vi "Chack Motor.vi"(11 "Input V70 Values":string) -> (0 "Low":string, 1 "High":string, 2 "Diff":string, 3 "diffAllowed":string, 4 "Result Motor Performance":string, 5 "Step Remark":string, 6 "error out":errorcluster, 7 "Status":bool)   [LabVIEW 2020, in "FBN_LATM.lvlib"]
uses:
  FBN_LATM.lvlib
  <vilib>/regexp/Match Regular Expression.xnode
panel:
  out "spreadsheet string":string
  out "Greater Than":bool
  out "OK?":bool
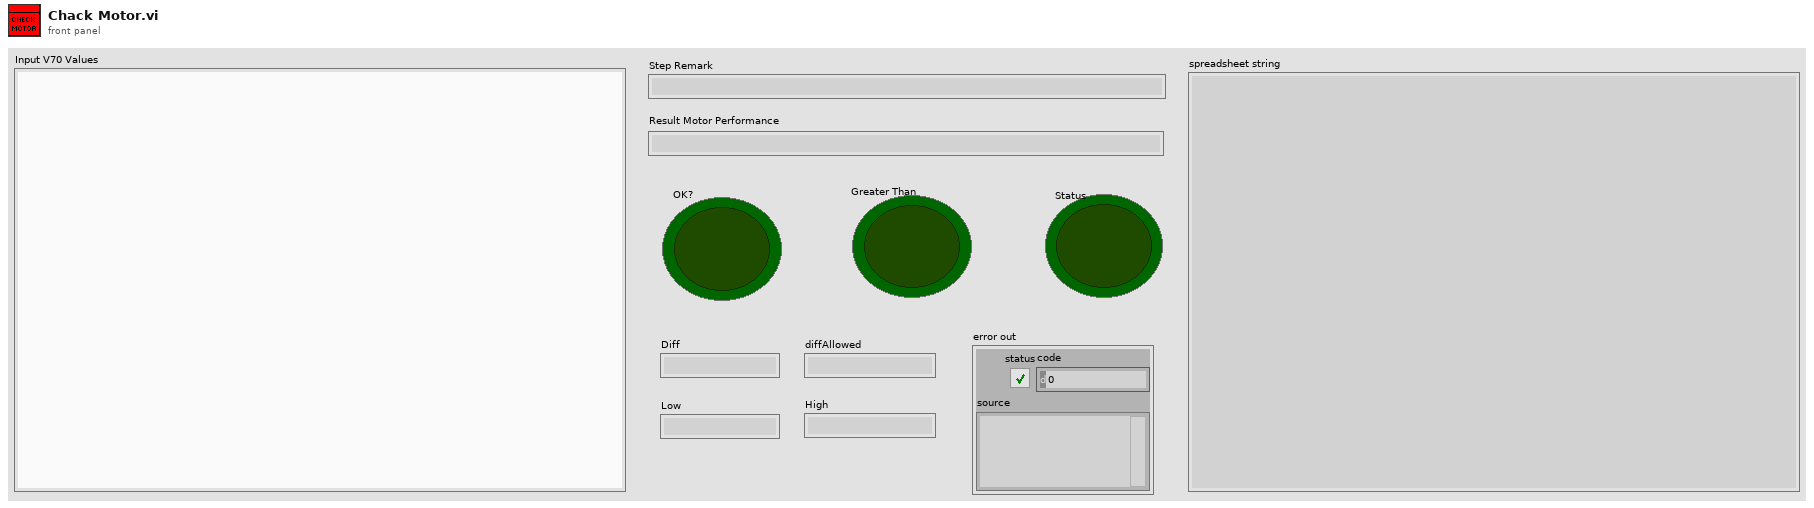
[diagram p1: front panel]
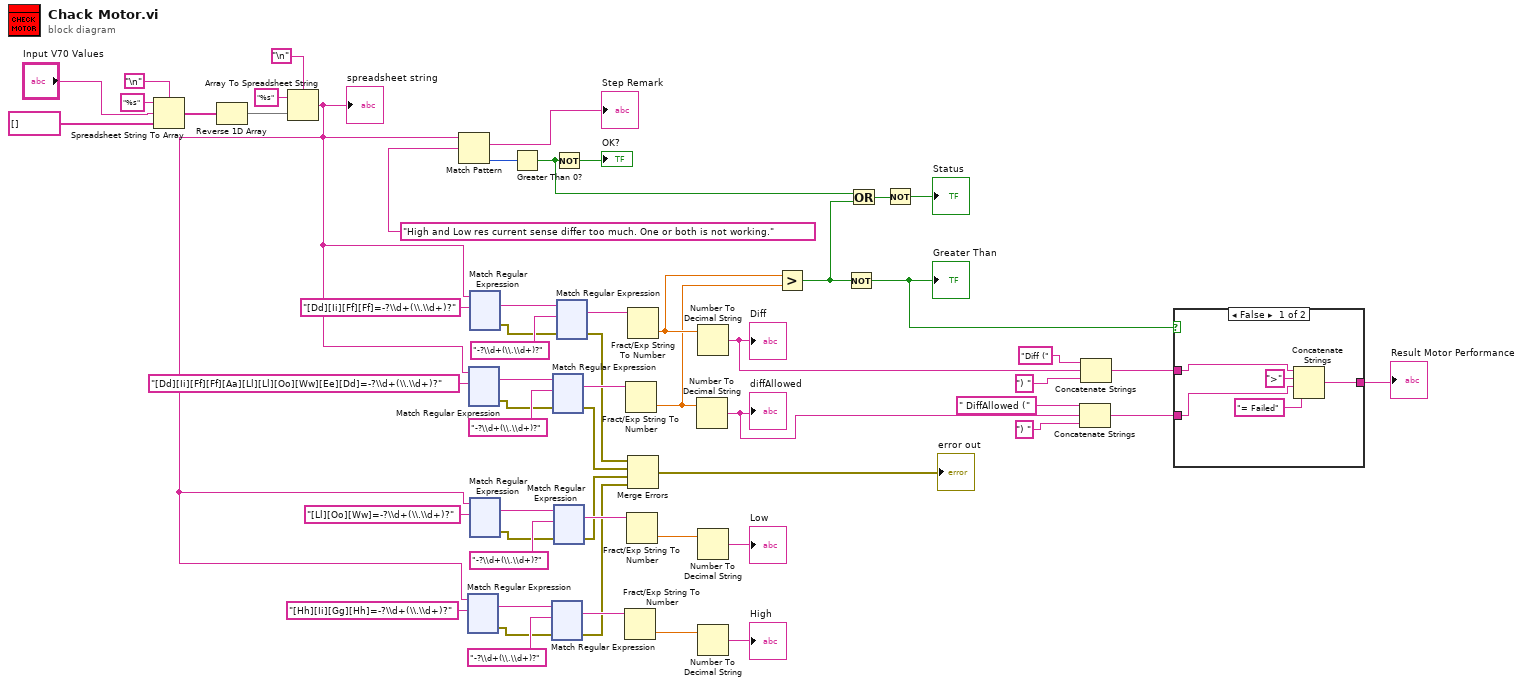
[diagram p0: block diagram]
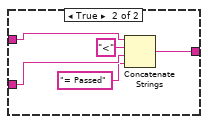
[diagram p2: hidden frame]
diagram:
  n1 = Spreadsheet String To Array(delimiter (Tab)="\n", format string="%s", spreadsheet string="Input V70 Values", array type (2D Dbl)=string[] []) -> (array=w17:string[])
  n2 = Reverse 1D Array(array=w17) -> (reversed array=w13:string[])
  n3 = Array To Spreadsheet String(delimiter (Tab)="\n", array=w13, 3:"%s" ("format string")) -> (spreadsheet string=w12:string)
  "spreadsheet string" <- w12
  n4 = Match Pattern(string=w12, regular expression="High and Low res current sense differ too much. One or both is not working.") -> (match substring=→"Step Remark":string, offset past match=w57:i32)  [unwired: 1 in, 2 out]
  n5 = xnode "Match Regular Expression"("input string"=w12, "regular expression"="[Hh][Ii][Gg][Hh]=-?\\d+(\\.\\d+)?") -> ("whole match"=w30:string, "error out"=w29:errorcluster)  [unwired: 4 in, 3 out]
  n6 = xnode "Match Regular Expression"("input string"=w12, "regular expression"="[Dd][Ii][Ff][Ff][Aa][Ll][Ll][Oo][Ww][Ee][Dd]=-?\\d+(\\.\\d+)?") -> ("whole match"=w48:string, "error out"=w46:errorcluster)  [unwired: 4 in, 3 out]
  n7 = xnode "Match Regular Expression"("input string"=w12, "regular expression"="[Dd][Ii][Ff][Ff]=-?\\d+(\\.\\d+)?") -> ("whole match"=w53:string, "error out"=w47:errorcluster)  [unwired: 4 in, 3 out]
  n8 = xnode "Match Regular Expression"("input string"=w12, "regular expression"="[Ll][Oo][Ww]=-?\\d+(\\.\\d+)?") -> ("whole match"=w35:string, "error out"=w34:errorcluster)  [unwired: 4 in, 3 out]
  n9 = Greater Than 0?(x=w57) -> (x > 0?=w40:bool)
  n10 = xnode "Match Regular Expression"("input string"=w30, "regular expression"="-?\\d+(\\.\\d+)?", "error in"=w29) -> ("whole match"=w31:string, "error out"=w27:errorcluster)  [unwired: 3 in, 3 out]
  n11 = xnode "Match Regular Expression"("input string"=w48, "regular expression"="-?\\d+(\\.\\d+)?", "error in"=w46) -> ("whole match"=w49:string, "error out"=w44:errorcluster)  [unwired: 3 in, 3 out]
  n12 = Not(x=w40) -> (.not. x?=→"OK?":bool)
  n13 = xnode "Match Regular Expression"("input string"=w35, "regular expression"="-?\\d+(\\.\\d+)?", "error in"=w34) -> ("whole match"=w36:string, "error out"=w28:errorcluster)  [unwired: 3 in, 3 out]
  n14 = xnode "Match Regular Expression"("input string"=w53, "regular expression"="-?\\d+(\\.\\d+)?", "error in"=w47) -> ("whole match"=w51:string, "error out"=w45:errorcluster)  [unwired: 3 in, 3 out]
  n15 = Fract/Exp String To Number(string=w31) -> (number=w22:dbl)  [unwired: 3 in, 1 out]
  n16 = Fract/Exp String To Number(string=w49) -> (number=w25:dbl)  [unwired: 3 in, 1 out]
  n17 = Fract/Exp String To Number(string=w36) -> (number=w21:dbl)  [unwired: 3 in, 1 out]
  n18 = Fract/Exp String To Number(string=w51) -> (number=w26:dbl)  [unwired: 3 in, 1 out]
  n19 = Merge Errors(w45, w44, w28, w27) -> (→"error out":errorcluster)
  n20 = Number To Decimal String(number=w25) -> (decimal integer string=w5:string)  [unwired: 1 in]
  "diffAllowed" <- w5
  n21 = Number To Decimal String(number=w26) -> (decimal integer string=w10:string)  [unwired: 1 in]
  "Diff" <- w10
  n22 = Number To Decimal String(number=w21) -> (decimal integer string=→"Low":string)  [unwired: 1 in]
  n23 = Number To Decimal String(number=w22) -> (decimal integer string=→"High":string)  [unwired: 1 in]
  n24 = Greater?(x=w26, y=w25) -> (0:w39:bool)
  n25 = Not(x=w39) -> (.not. x?=w1:bool)
  "Greater Than" <- w1
  n26 = Or(x=w40, y=w39) -> (x .or. y?=w41:bool)
  n27 = Not(x=w41) -> (.not. x?=→"Status":bool)
  n28 = Concatenate Strings(" DiffAllowed (", w5, ") " ("string")) -> (w3:string)
  n29 = Concatenate Strings("Diff (", w10, ") " ("string")) -> (w4:string)
  n30 = case shown="False" w1 {
    tunnel: w4 -> [w63 w67]
    tunnel: w3 -> [w61 w66]
    tunnel: [w59 w64] -> w2
    frame False {
      n31 = Concatenate Strings(w63, ">" ("string"), w61, "= Failed" ("string")) -> (w59:string)
    }
    frame True {
      n32 = Concatenate Strings(w67, "<" ("string"), w66, "= Passed" ("string")) -> (w64:string)
    }
  }
  "Result Motor Performance" <- w2
